vi "SetVerbosity.vi"(8 "error in (no error)":errorcluster, 11 "Verbosity":T1) -> (0 "error out":errorcluster)   [LabVIEW 2026, in "Lumberjack.lvlib"]
doc: "Writes the process CatchError verbosity into the process-global store.\nSets the single-element queue keyed \"ProcessCatchErrorVerbosity\"; written by ConfigureVerbosity and read by CatchError to gate its dialog.\nLumberjack.lvlib, private (library-internal)."
uses:
  Lumberjack.lvlib
  TypeDefs/Severity.ctl
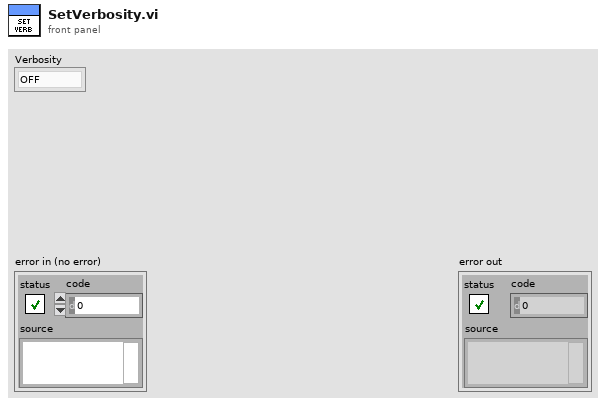
[diagram p1: front panel]
types:
  T1 = typedef "Lumberjack.lvlib/Severity.ctl" = enum16{"OFF", "FATAL", "ERROR", "WARN", "INFO", "DEBUG", "TRACE", "ALL"}
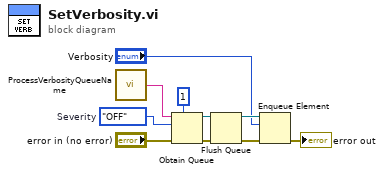
[diagram p0: block diagram]
diagram:
  w3 = Severity."OFF"  # Severity
  n1 = call "ProcessVerbosityQueueName.vi"() -> ("processVerbosityQueueName"=w6:string)
  n2 = Obtain Queue(max queue size (-1, unlimited)=1, name (unnamed)=w6, element data type=w3, error in (no error)="error in (no error)") -> (queue out=w7:refnum<queue>, error out=w9:errorcluster)  [unwired: 1 in, 1 out]
  n3 = Flush Queue(queue=w7, error in (no error)=w9) -> (queue out=w2:refnum<queue>, error out=w5:errorcluster)  [unwired: 1 out]
  n4 = Enqueue Element(queue=w2, element="Verbosity", error in (no error)=w5) -> (error out=→"error out":errorcluster)  [unwired: 1 in, 2 out]
